vi "LoadButtons.vi"(4 "SubPanel Command":T1, 5 "MenuButtons":path[](array[path]), 6 "error in (no error)":errorcluster, 7 "SubMenuButtons":path[](array[path]), 8 "SubMenuButtonVIs":refnum<vi>[](array[refnum]), 9 "MenuButtonVIs":refnum<vi>[](array[refnum])) -> (0 "error out":errorcluster)   [LabVIEW 2023]
uses:
  ButtonCommands.ctl
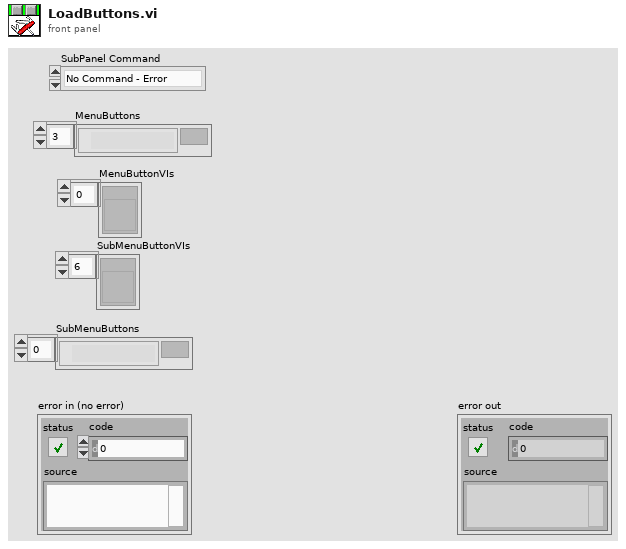
[diagram p1: front panel]
types:
  T1 = typedef "ButtonCommands.ctl" = enum16{"No Command - Error", "Load Buttons", "Remove Buttons"}
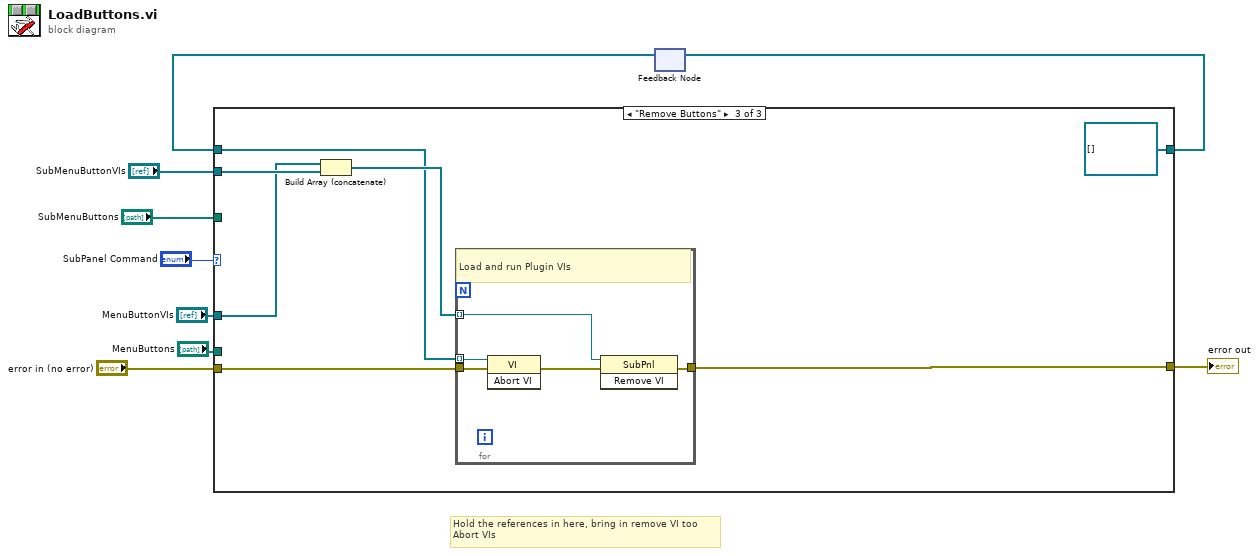
[diagram p0: block diagram]
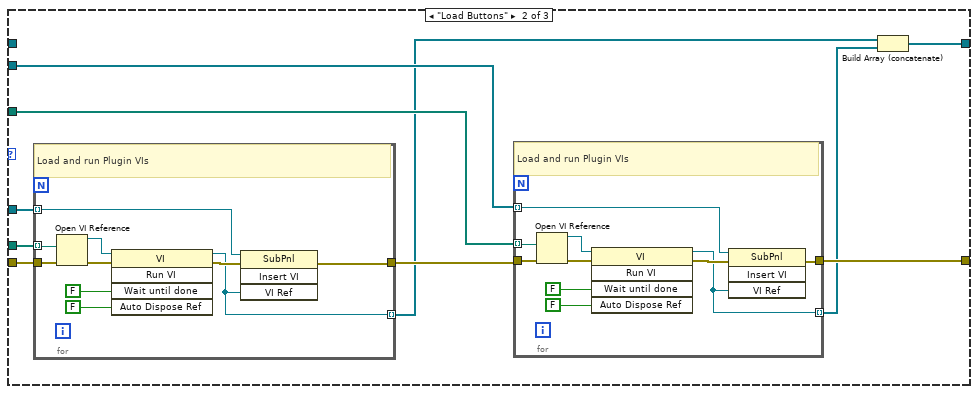
[diagram p3: hidden frame]
diagram:
  # "Hold the references in here, bring in remove VI too\nAbort VIs"
  n1 = feedback #1() -> (w1:refnum<vi>[])  [unwired: 1 in]
  n2 = case shown="\"Remove Buttons\"" "SubPanel Command" {
    tunnel: "MenuButtons" -> [_ w21 _]
    tunnel: "error in (no error)" -> [w10 w20 w47]
    tunnel: "MenuButtonVIs" -> [_ w19 w43]
    tunnel: [w10 w18 w48] -> w6
    tunnel: "SubMenuButtonVIs" -> [_ w16 w46]
    tunnel: "SubMenuButtons" -> [_ w15 _]
    tunnel: [w11 w12 refnum<vi>[] []] -> w2
    tunnel: w1 -> [w11 _ w42]
    frame "No Command - Error", Default {
    }
    frame "Load Buttons" {
      n3 = for {
        tunnel: w20 -> [w37]
        tunnel: [w34] -> w17
        tunnel: w21 -> [w36] mode=indexing
        tunnel: w19 -> [w33] mode=indexing
        tunnel: [w32] -> w14 mode=indexing
        # "Load and run Plugin VIs"
        n4 = Open VI Reference(vi path=w36, error in (no error)=w37) -> (vi reference=w38:refnum<vi>, error out=w39:errorcluster)  [unwired: 4 in]
        n5 = invoke class="VI" method="Run VI"(reference=w38, error in=w39, "Wait until done"=FALSE ("Wait Until Done"), "Auto Dispose Ref"=FALSE ("Auto Dispose Reference")) -> (reference out=w32:refnum<vi>, error out=w35:errorcluster)  [unwired: 1 in, 3 out]
        n6 = invoke on="Invoke Node" class="SubPnl" method="Insert VI"(reference=w33, error in=w35, "VI Ref"=w32) -> (error out=w34:errorcluster)  [unwired: 1 in, 3 out]
      }
      n7 = for {
        tunnel: w17 -> [w27]
        tunnel: [w24] -> w18
        tunnel: w15 -> [w26] mode=indexing
        tunnel: w16 -> [w23] mode=indexing
        tunnel: [w22] -> w13 mode=indexing
        # "Load and run Plugin VIs"
        n8 = Open VI Reference(vi path=w26, error in (no error)=w27) -> (vi reference=w28:refnum<vi>, error out=w29:errorcluster)  [unwired: 4 in]
        n9 = invoke class="VI" method="Run VI"(reference=w28, error in=w29, "Wait until done"=FALSE ("Wait Until Done"), "Auto Dispose Ref"=FALSE ("Auto Dispose Reference")) -> (reference out=w22:refnum<vi>, error out=w25:errorcluster)  [unwired: 1 in, 3 out]
        n10 = invoke on="Invoke Node" class="SubPnl" method="Insert VI"(reference=w23, error in=w25, "VI Ref"=w22) -> (error out=w24:errorcluster)  [unwired: 1 in, 3 out]
      }
      n11 = Build Array (concatenate)(w14, w13) -> (w12:refnum<vi>[])
    }
    frame "Remove Buttons" {
      n12 = Build Array (concatenate)(w43, w46) -> (w44:refnum<vi>[])
      n13 = for {
        tunnel: w47 -> [w50]
        tunnel: [w52] -> w48
        tunnel: w42 -> [w49] mode=indexing
        tunnel: w44 -> [w51] mode=indexing
        # "Load and run Plugin VIs"
        n14 = invoke class="VI" method="Abort VI"(reference=w49, error in=w50) -> (error out=w53:errorcluster)  [unwired: 1 in, 2 out]
        n15 = invoke on="Invoke Node" class="SubPnl" method="Remove VI"(reference=w51, error in=w53) -> (error out=w52:errorcluster)  [unwired: 1 in, 2 out]
      }
    }
  }
  "error out" <- w6
  n16 = feedback-in #1(w2) -> ()
